vi "CANOpen_NMT_Setup HB.vi"(7 "Node ID":u8, 8 "error in":errorcluster, 10 "Period":u16, 11 "interface object in":refnum<k20>) -> (0 "error out":errorcluster, 3 "interface object out":refnum<k20>)   [LabVIEW 2021, in "CANOpen Addon Engine.lvlib"]
uses:
  <vilib>/CANopenLib/CANOPEN.llb/CANopen SDO Create.vi
  <vilib>/CANopenLib/CANOPEN.llb/CANopen SDO Write [U16].vi
  <vilib>/CANopenLib/CANOPEN.llb/CANopen SDO Close.vi
  CANOpen Addon Engine.lvlib
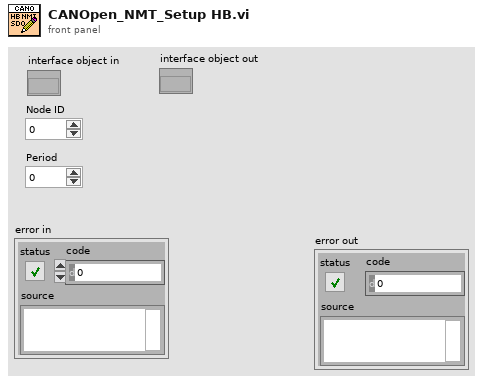
[diagram p1: front panel]
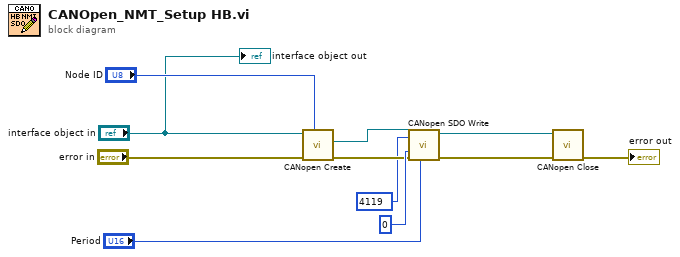
[diagram p0: block diagram]
diagram:
  n1 = call-poly <vilib>:"CANopen Create.vi"("node-ID"="Node ID", "error in (no error)"="error in", "interface object in"="interface object in") -> ("error out"=w6:errorcluster, "SDO object out"=w5:refnum<k20>)  [unwired: 6 in, 1 out]
  n2 = call-poly <vilib>:"CANopen SDO Write.vi"("U16 data"="Period", "error in (no error)"=w6, "object sub-index (0)"=u8 0, "object index"=u16 4119, "SDO object in"=w5) -> ("error out"=w2:errorcluster, "SDO object out"=w3:refnum<k20>)  [unwired: 4 in, 1 out]
  n3 = call-poly <vilib>:"CANopen Close.vi"("error in (no error)"=w2, "SDO object in"=w3) -> ("error out"=→"error out":errorcluster)  [unwired: 9 in]
  "interface object out" <- "interface object in"
